vi "BMark_Save Tokens.vi"(10 "reference":refnum<vi>, 11 "GroupByVI":bool) -> ()   [LabVIEW 2017]
uses:
  <resource>/dialog/lvconfig.llb/LV Config Write String.vi
  <resource>/dialog/lvconfig.llb/LV Config Write Boolean.vi
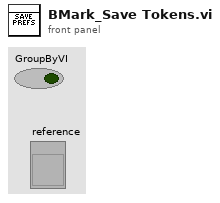
[diagram p1: front panel]
types:
  T1 = typedef "LVRectTypeDef.ctl" = cluster{"Left":i16, "Top":i16, "Right":i16, "Bottom":i16}
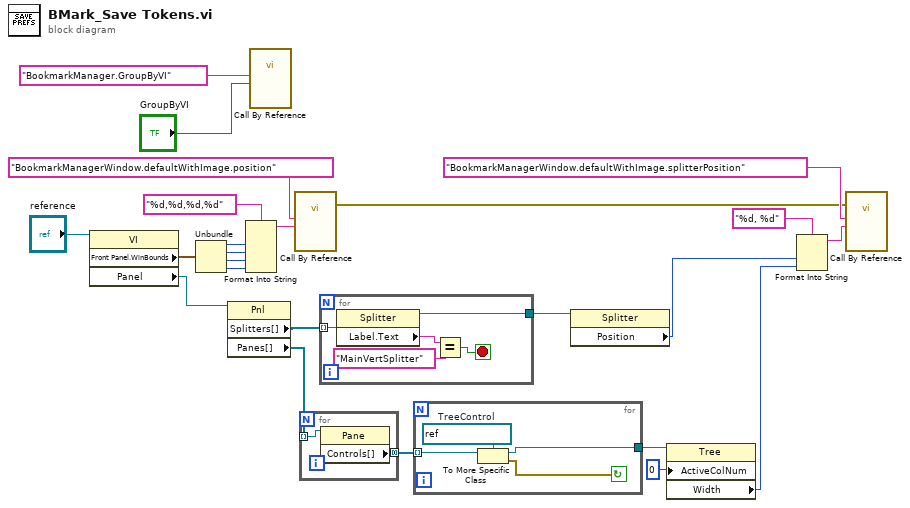
[diagram p0: block diagram]
diagram:
  n1 = property class="VI"(reference="reference") -> ("Front Panel.WinBounds"=w23:T1, "Panel"=w13:refnum<vi>)  [unwired: 1 in, 2 out]
  n2 = Unbundle(w23) -> ("Left"=w17:i16, "Top"=w18:i16, "Right"=w19:i16, "Bottom"=w20:i16)
  n3 = property class="Pnl"(reference=w13) -> ("Splitters[]"=w12:refnum<vi>[], "Panes[]"=w6:refnum<vi>[])  [unwired: 1 in, 2 out]
  n4 = Format Into String(format string="%d,%d,%d,%d", w17, w18, w19, w20) -> (resulting string=w22:string)  [unwired: 2 in, 1 out]
  n5 = call-by-ref "?"("value"="GroupByVI", "key"="BookmarkManager.GroupByVI") -> ()  [unwired: 7 in, 3 out]
  n6 = call-by-ref "?"("value"=w22, "key"="BookmarkManagerWindow.defaultWithImage.position") -> (error out=w8:errorcluster)  [unwired: 3 in, 6 out]
  n7 = for {
    tunnel: w6 -> [w26] mode=indexing
    tunnel: [w25] -> w5 mode=concatenating
    n8 = property class="Pane"(reference=w26) -> ("Controls[]"=w25:refnum<vi>[])  [unwired: 1 in, 2 out]
  }
  n9 = for {
    tunnel: w12 -> [w31] mode=indexing
    tunnel: [w28] -> w11
    stop <- w27 stop-if-true
    n10 = property class="Splitter"(reference=w31) -> (reference out=w28:refnum<vi>, "Label.Text"=w30:string)  [unwired: 1 in, 1 out]
    n11 = Equal?(x=w30, y="MainVertSplitter") -> (x = y?=w27:bool)
  }
  n12 = for {
    tunnel: [w34] -> w2
    tunnel: w5 -> [w33] mode=indexing
    stop <- w32 continue-if-true
    w35 = refnum<vi> refnum  # TreeControl
    n13 = To More Specific Class(target class=w35, reference=w33) -> (specific class reference=w34:refnum<vi>, error out=w32:errorcluster)  [unwired: 1 in]
  }
  n14 = property class="Splitter"(reference=w11) -> ("Position"=w7:i32)  [unwired: 1 in, 2 out]
  n15 = property class="Tree"(reference=w2, "ActiveColNum"=0 ("Active Cell:Active Column Number")) -> ("Width"=w1:i32)  [unwired: 1 in, 2 out]
  n16 = Format Into String(format string="%d, %d", w7, w1) -> (resulting string=w4:string)  [unwired: 2 in, 1 out]
  n17 = call-by-ref "?"(error in=w8, "value"=w4, "key"="BookmarkManagerWindow.defaultWithImage.splitterPosition") -> ()  [unwired: 2 in, 7 out]
